vi "Top Level FPGA_w8randLED.vi"() -> ()   [LabVIEW 2012]
uses:
  <vilib>/Platform/TimedLoop/XDataNode/timing_clust.ctl
  <vilib>/Platform/TimedLoop/XDataNode/nitl_modes.ctl
  <vilib>/Platform/TimedLoop/XDataNode/wakeup.ctl
  <vilib>/rvi/DataTransferAndStorage/Container/Common/niFpgaContainerMetaDataKey.ctl
  <vilib>/rvi/DataTransferAndStorage/Container/Common/niFpgaContainerState.ctl
  <vilib>/rvi/DataTransferAndStorage/Container/Common/niFpgaDataTypeControl.ctl
  <vilib>/rvi/DataTransferAndStorage/Container/Common/niFpgaContainerImplementationControl.ctl
  <vilib>/rvi/DataTransferAndStorage/Container/Common/niFpgaContainerArbitrationOptionsControl.ctl
  <vilib>/rvi/DataTransferAndStorage/Container/Common/niFpgaTransferTypeControl.ctl
  <vilib>/rvi/DataTransferAndStorage/Container/Common/niFpgaContainerInitializationParameters.ctl
  <vilib>/rvi/Memory/Memory_Types/niFpgaMemoryInterfaceConfiguration.ctl
  <vilib>/rvi/FIFO/Fifo_Types/niFpgaFifoControlLogicControl.ctl
  <vilib>/rvi/eio/common/nirviEmuTemplateMethod_errors.vi
  <vilib>/rvi/FIFO/Fifo_Resource/nirvififoEmulationSetSize.vi
  <vilib>/rvi/DataTransferAndStorage/Container/Common/niFpgaContainerGetUniqueNameForEmu.vi
  <vilib>/rvi/Emulation/niFpgaSctlEmulationRegisterWithScheduler.vi
  <vilib>/rvi/DataTransferAndStorage/Container/Common/niFpgaContainerSetEmuInfo.vi
  <vilib>/rvi/eio/common/nirviEmuReportErrorAndStop.vi
  <vilib>/rvi/Emulation/niFpgaSctlEmulationScheduler.vi
  <vilib>/rvi/Emulation/niFpgaSctlEmulationFifoFullMgr.vi
  <vilib>/rvi/errors/niFpgaSetErrorForExecOnDevCompSimple.vi
  <vilib>/rvi/Memory/Memory_Emulation/nirvimemoryEmulationManagerCache_GetValue.vi
  <vilib>/rvi/Memory/Memory_Emulation/niFpgaMemoryEmulationValidateCache.vi
  <vilib>/rvi/Memory/Memory_Emulation/nirvimemoryEmulationManagerCache_InsertValue.vi
  <vilib>/rvi/Memory/Memory_Emulation/nirvimemoryEmulationManagerCache_SetValue.vi
  <vilib>/rvi/Emulation/niFpgaSctlEmulationResourceMgr.vi
  <vilib>/rvi/Memory/Memory_Emulation/niFpgaMemoryEmulationCacheClearOnFirstRun.vi
  <vilib>/rvi/Memory/Memory_Emulation/nirvimemoryEmulationManagerCache_MakeExclusive.vi
  <vilib>/rvi/Memory/Memory_Emulation/nirvimemoryEmulationManagerCache_ReleaseExclusive.vi
  <vilib>/Utility/error.llb/Clear Errors.vi
  <vilib>/eio/EIONode/EIONode.xnode
  <vilib>/rvi/DataTransferAndStorage/Container/XNode/niFpgaContainer.xnode
  <vilib>/rvi/FIFO/Fifo_Resource/nirvififoEmulationClear.vi
  <vilib>/Platform/TimedLoop/XDataNode/XDataNode.xnode
  <vilib>/rvi/LocalResourceManager/LocalResourceManager.xnode
  <vilib>/rvi/FIFO/Fifo_Resource/nirvififoEmulationRead.vi
  <vilib>/rvi/DataTransferAndStorage/Register/Emulation/niFpgaRegisterEmulation.vi
  <vilib>/rvi/Memory/Memory_Emulation/nirvimemoryEmulation.vi
  <vilib>/rvi/FIFO/Fifo_Resource/nirvififoEmulationWrite.vi
  <vilib>/Platform/TimedLoop/XDataNode/XDNodeRunTimeDep.lvlib
panel:
  in  "location":i16(ring) items=["Purdue", "NIKHEF", "Zurich", "???"]
  in  "Testpulse duration (20 ns ticks)":u32=5
  in  "channel 7 on/off":bool
  in  "channel 6 on/off":bool
  in  "channel 5 on/off":bool
  in  "channel 4 on/off":bool
  in  "channel 3 on/off":bool
  in  "channel 1 on/off":bool
  in  "channel 2 on/off":bool
  in  "channel 0 on/off":bool
  out "Timestamp":u64
  in  "Stop FPGA and exit":bool
  out "DMA FIFO Timed Out?":bool
  in  "Testpulser On/Off":bool
  in  "Testpulse Time Delay (20 ns ticks)":u32=14
  in  "circular buffer length":u32=1000
  in  "# of pretrigger":u32=20
  out "IO Module\\Pll Unlocked":bool
  out "IO Module\\ADC Error B":bool
  out "IO Module\\ADC Error A":bool
  out "Init Done":bool
  in  "Trigger 4":i16=4000
  in  "Trigger 5":i16=4000
  in  "Trigger 6":i16=4000
  in  "Trigger 7":i16=4000
  in  "Trigger 2":i16=4000
  in  "Trigger 3":i16=4000
  in  "Trigger 1":i16=4000
  in  "Record Size only data":u32=95
  in  "Trigger 0":i16=4000
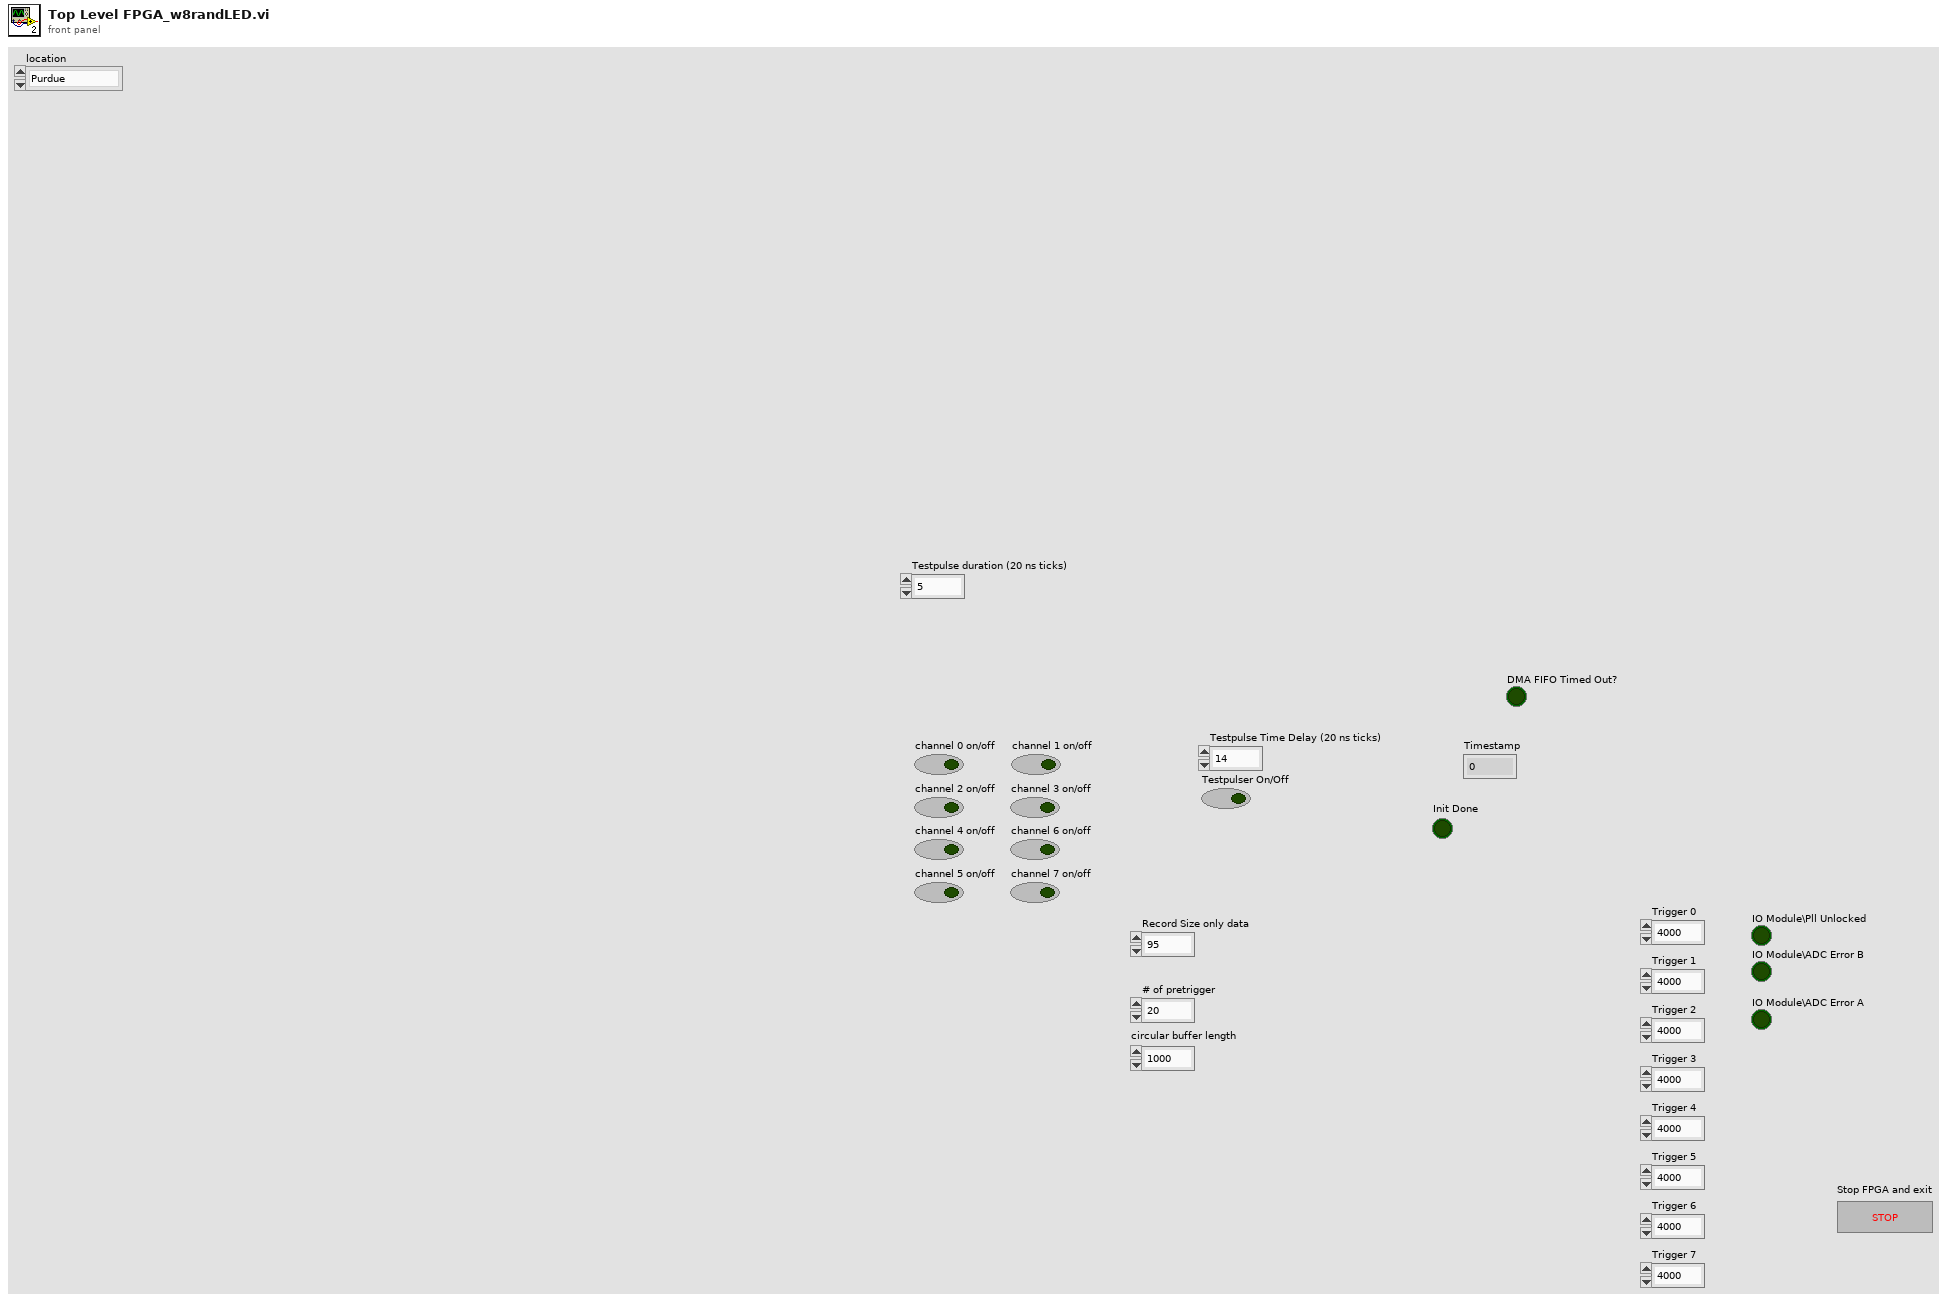
[diagram p1: front panel]
types:
  T1 = typedef "XDNodeRunTimeDep.lvlib/timing_clust.ctl" = cluster{"Expected End [f-1]":u64, "Actual End [f-1]":u64, "Finished Late? [f-1]":bool, "Expected End [i-1]":u64, "Actual End [i-1]":u64, "Finished Late? [i-1]":bool, "Expected Start [i]":u64, "Actual Start [i]":u64, "Expected Start [f]":u64, "Actual Start [f]":u64, "Source Name":string, "Structure Name":string, "Period":i64, "Deadline":i64, "Offset":i64, "Start":i64, "Priority":i32, "Timeout":i32, "Mode":T2, "Wakeup Reason":T3, "Error":errorcluster, "Source Type":string, "Secondary Source Type":string, "Global End Time":u64, "Global Start Time":u64, "Frame Duration":u64, "Iteration Duration":u64, "Assigned CPU":i32, "I/O Scan Engine Mode":u32}
  T2 = typedef "XDNodeRunTimeDep.lvlib/nitl_modes.ctl" = enum32{"No Change", "Process missed periods, maintain original phase", "Discard missed periods, maintain original phase", "Process missed periods, ignore original phase", "Discard missed periods, ignore original phase"}
  T3 = typedef "XDNodeRunTimeDep.lvlib/wakeup.ctl" = enum32{"Normal", "Aborted", "Asynchronous wakeup", "Timing source error", "Timed loop error", "Timeout"}
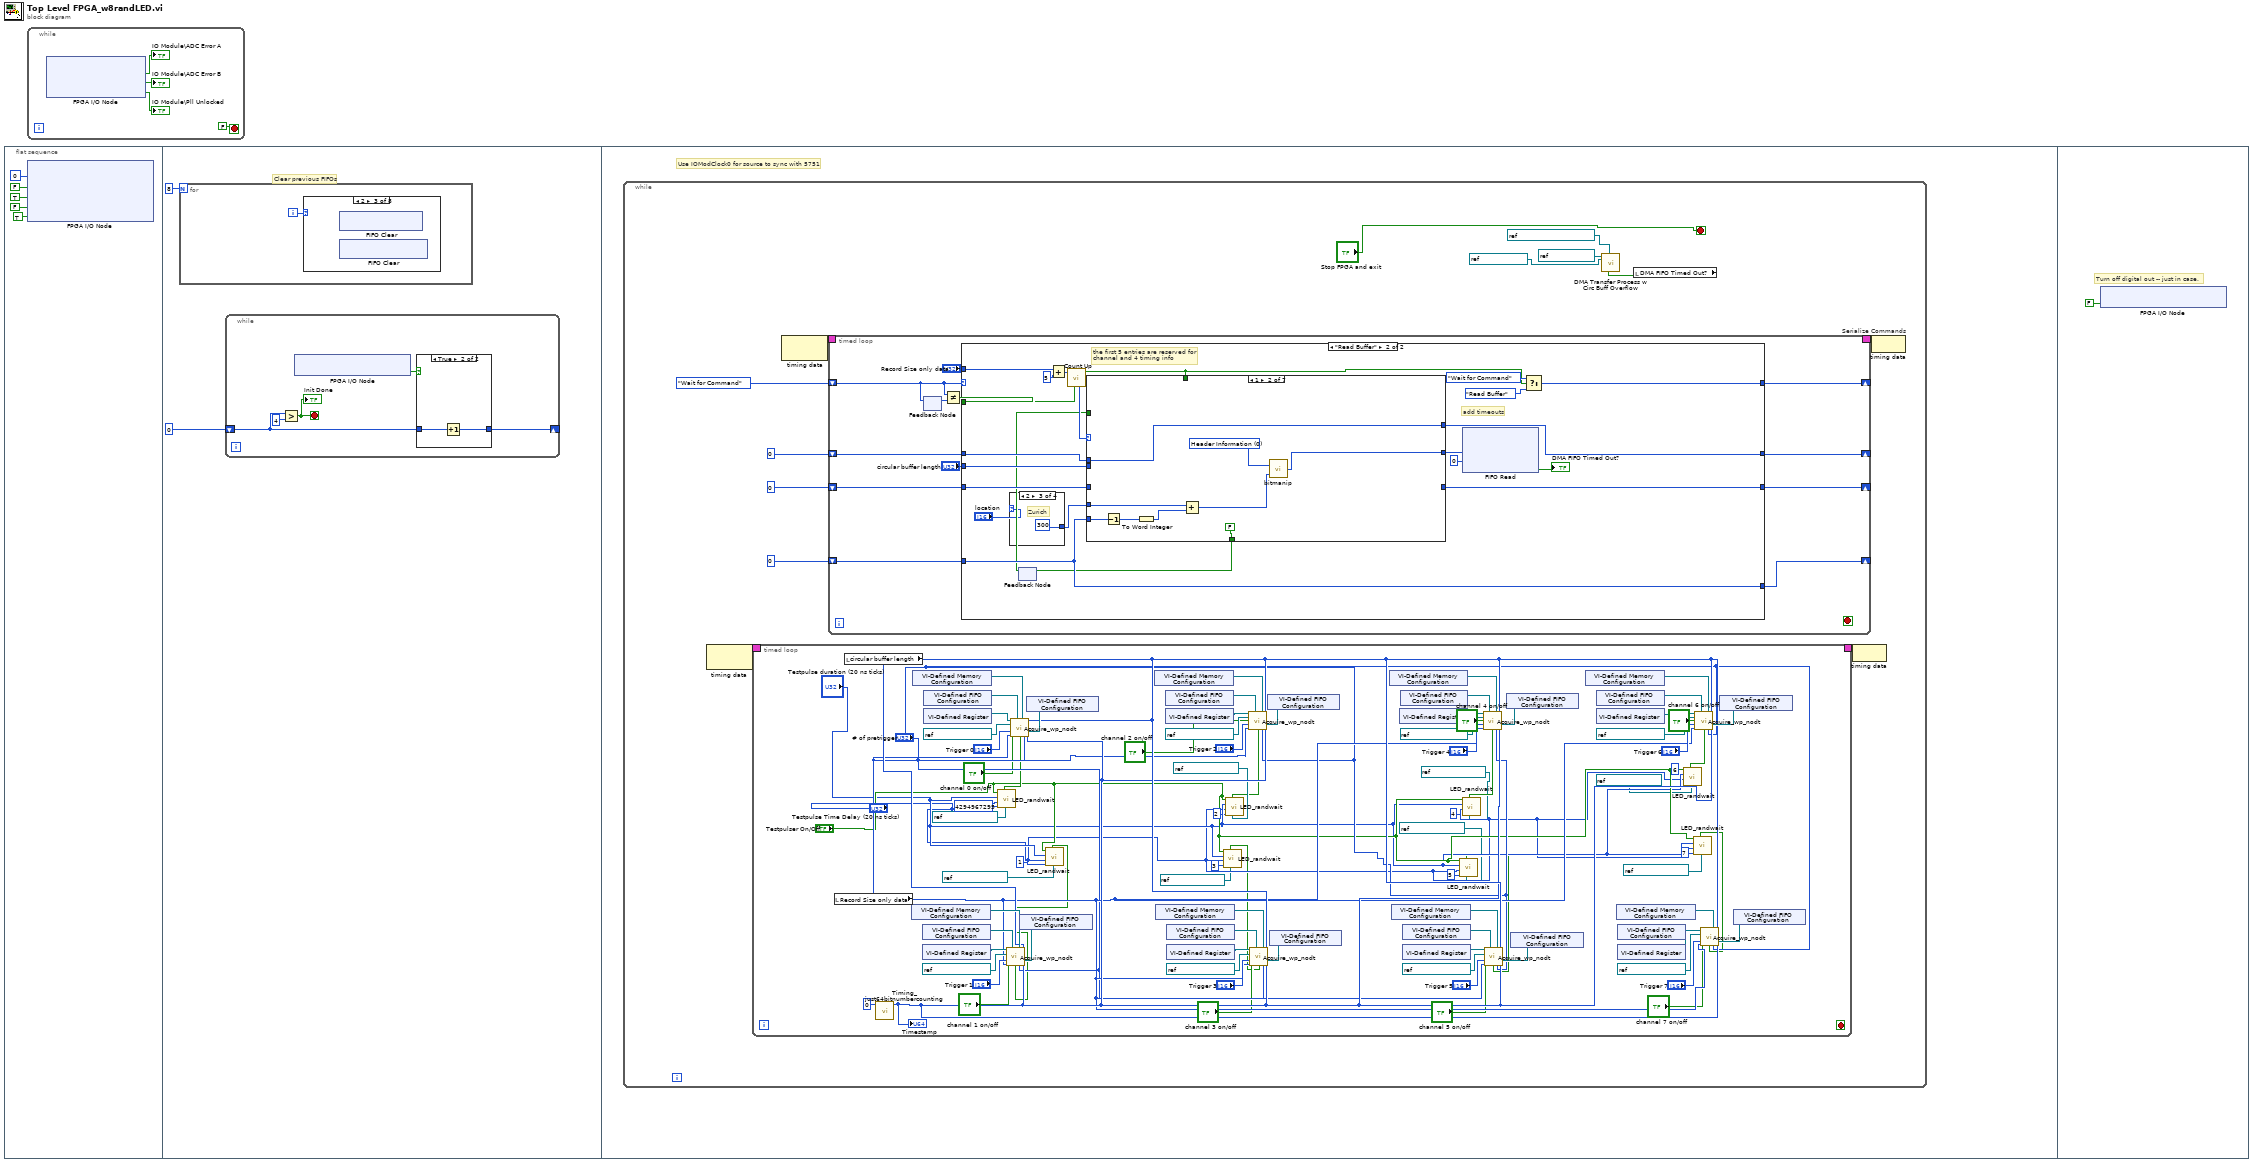
[diagram p0: block diagram]
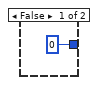
[diagram p2: hidden frame]
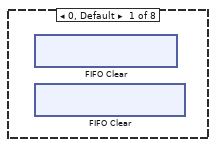
[diagram p3: hidden frame]
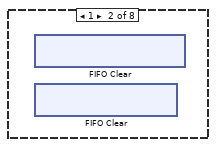
[diagram p4: hidden frame]
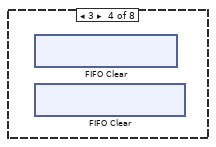
[diagram p5: hidden frame]
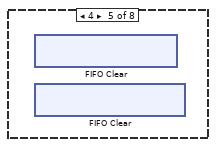
[diagram p6: hidden frame]
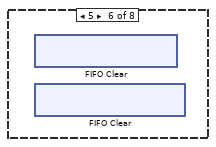
[diagram p7: hidden frame]
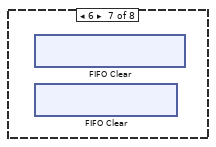
[diagram p8: hidden frame]
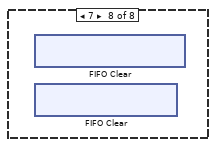
[diagram p9: hidden frame]
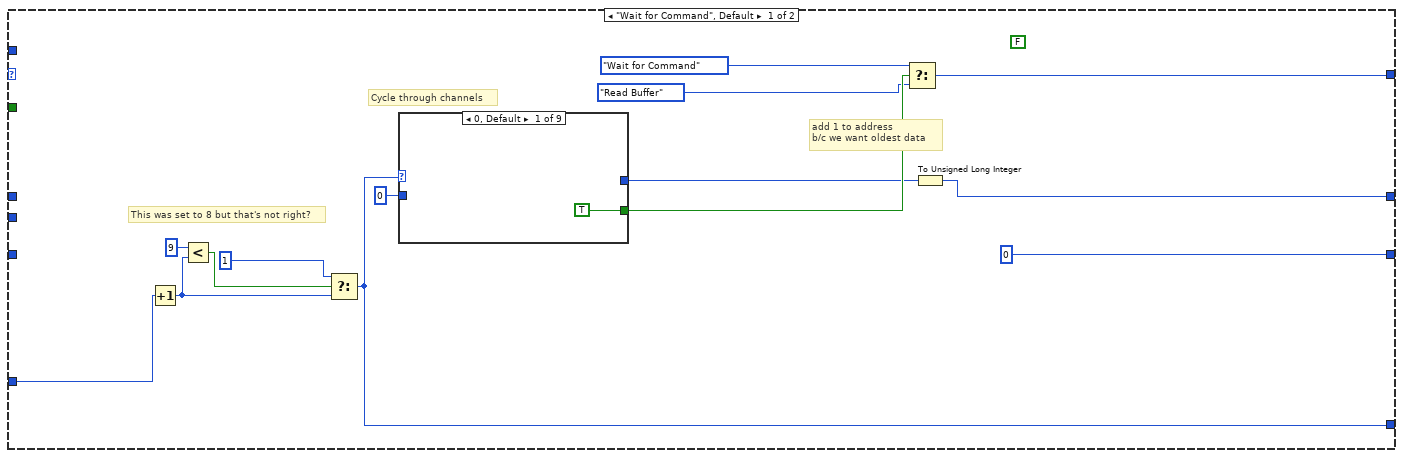
[diagram p10: hidden frame]
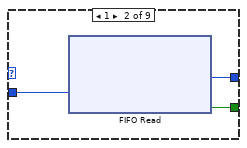
[diagram p11: hidden frame]
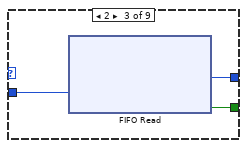
[diagram p12: hidden frame]
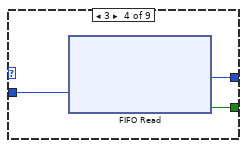
[diagram p13: hidden frame]
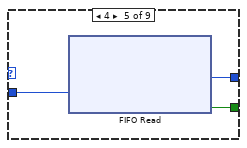
[diagram p14: hidden frame]
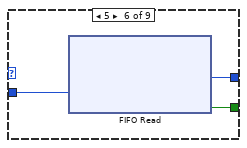
[diagram p15: hidden frame]
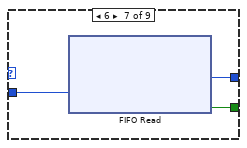
[diagram p16: hidden frame]
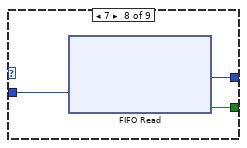
[diagram p17: hidden frame]
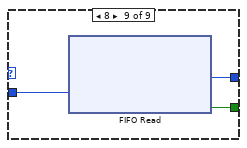
[diagram p18: hidden frame]
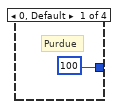
[diagram p19: hidden frame]
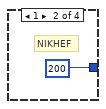
[diagram p20: hidden frame]
diagram:
  n1 = flat-sequence {
    frame #0 {
      n2 = xnode "FPGA I/O Node"("IO Module\\Sample Clock Select"=u8 0 ("IO Module\\Sample Clock Select"), "IO Module\\Force Initialization"=FALSE ("IO Module\\Force Initialization"), "IO Module\\Force Initialization"=TRUE ("IO Module\\Force Initialization"), "IO Module\\Force Initialization"=FALSE ("IO Module\\Force Initialization"), "IO Module\\Digital Output Enable"=TRUE ("IO Module\\Digital Output Enable")) -> ()  [unwired: 5 in, 5 out]
    }
    frame #1 {
      # "Clear previous FIFOs"
      n3 = for {
        N: 8 -> [_]
        i -> [w16]
        n4 = case shown="2" w16 {
          frame 0, Default {
            n5 = xnode ("FIFO Clear")() -> ()  [unwired: 1 in, 1 out]
            n6 = xnode ("FIFO Clear")() -> ()  [unwired: 1 in, 1 out]
          }
          frame 1 {
            n7 = xnode ("FIFO Clear")() -> ()  [unwired: 1 in, 1 out]
            n8 = xnode ("FIFO Clear")() -> ()  [unwired: 1 in, 1 out]
          }
          frame 2 {
            n9 = xnode ("FIFO Clear")() -> ()  [unwired: 1 in, 1 out]
            n10 = xnode ("FIFO Clear")() -> ()  [unwired: 1 in, 1 out]
          }
          frame 3 {
            n11 = xnode ("FIFO Clear")() -> ()  [unwired: 1 in, 1 out]
            n12 = xnode ("FIFO Clear")() -> ()  [unwired: 1 in, 1 out]
          }
          frame 4 {
            n13 = xnode ("FIFO Clear")() -> ()  [unwired: 1 in, 1 out]
            n14 = xnode ("FIFO Clear")() -> ()  [unwired: 1 in, 1 out]
          }
          frame 5 {
            n15 = xnode ("FIFO Clear")() -> ()  [unwired: 1 in, 1 out]
            n16 = xnode ("FIFO Clear")() -> ()  [unwired: 1 in, 1 out]
          }
          frame 6 {
            n17 = xnode ("FIFO Clear")() -> ()  [unwired: 1 in, 1 out]
            n18 = xnode ("FIFO Clear")() -> ()  [unwired: 1 in, 1 out]
          }
          frame 7 {
            n19 = xnode ("FIFO Clear")() -> ()  [unwired: 1 in, 1 out]
            n20 = xnode ("FIFO Clear")() -> ()  [unwired: 1 in, 1 out]
          }
        }
      }
      n21 = while {
        shift-right: [w11] -> _
        shift-left: u16 0 -> [w10]
        stop <- w8 stop-if-true
        n22 = Greater?(x=w10, y=u16 4) -> (0:w8:bool)
        "Init Done" <- w8
        n23 = xnode "FPGA I/O Node"() -> ("IO Module\\Initialization Done"=w12:bool)  [unwired: 1 in, 1 out]
        n24 = case shown="True" w12 {
          tunnel: [u16 0 w15] -> w11
          tunnel: w10 -> [_ w14]
          frame False {
          }
          frame True {
            n25 = Increment(x=w14) -> (x+1=w15:u16)
          }
        }
      }
    }
    frame #2 {
      # "Use IOModClock0 for source to sync with 5751"
      n26 = while {
        stop <- "Stop FPGA and exit" stop-if-true
        n27 = node-c288() -> (w22:T1)  [unwired: 1 in]
        n28 = timed-loop {
          timing: w22 -> [_]
          timing-out: [_] -> w21
          stop <- _ stop-if-true
          n29 = local read "Record Size only data"() -> (w68:u32)
          n30 = local read "circular buffer length"() -> (w70:u32)
          n31 = call "Timing_just64bitnumbercounting.vi"("initial value"=u64 0) -> ("x+1"=w69:u64)  [unwired: 10 in]
          "Timestamp" <- w69
          n32 = xnode "VI-Defined Memory Configuration"() -> ("Memory Out"=w116:refnum<k21>)
          n33 = xnode "VI-Defined Memory Configuration"() -> ("Memory Out"=w71:refnum<k21>)
          n34 = xnode "VI-Defined FIFO Configuration"() -> ("FIFO Out"=w115:refnum<k21>)
          n35 = xnode "VI-Defined Register"() -> ("Register Out"=w96:refnum<k21>)
          n36 = xnode "VI-Defined FIFO Configuration"() -> ("FIFO Out"=w72:refnum<k21>)
          n37 = xnode "VI-Defined Register"() -> ("Register Out"=w67:refnum<k21>)
          n38 = call "LED_randwait.vi"("FPGA I/O In"=refnum<k21> "IO Module\\D0 0", "seed"=u32 4294967295, "Testpulse Time Delay (20 ns ticks)"="Testpulse Time Delay (20 ns ticks)", "Testpulse duration (20 ns ticks)"="Testpulse duration (20 ns ticks)", "Testpulser On/Off"="Testpulser On/Off") -> ("Is Test Pulse?"=w56:bool)  [unwired: 5 in, 1 out]
          n39 = xnode "VI-Defined FIFO Configuration"() -> ("FIFO Out"=w82:refnum<k21>)
          n40 = xnode "VI-Defined FIFO Configuration"() -> ("FIFO Out"=w75:refnum<k21>)
          n41 = call "Acquire_wp_nodt.vi"("Ch Armed Reg"=w67, "Command FIFO"=w72, "Circular Buffer Mem"=w71, "circular buffer length"=w70, "FPGA I/O In"=refnum<k21> "IO Module\\AI A0", "channel on/off"="channel 0 on/off", "Trigger"="Trigger 0", "Timing FIFO"=w75, "Samples to Acquire"=w68, "Is Test Pulse?"=w56, "# of pretrigger"="# of pretrigger", "timing"=w69) -> ()  [unwired: 4 in]
          n42 = call "LED_randwait.vi"("FPGA I/O In"=refnum<k21> "IO Module\\D0 1", "seed"=u32 1, "Testpulse Time Delay (20 ns ticks)"="Testpulse Time Delay (20 ns ticks)", "Testpulse duration (20 ns ticks)"="Testpulse duration (20 ns ticks)", "Testpulser On/Off"="Testpulser On/Off") -> ("Is Test Pulse?"=w55:bool)  [unwired: 5 in, 1 out]
          n43 = call "Acquire_wp_nodt.vi"("Ch Armed Reg"=w96, "Command FIFO"=w115, "Circular Buffer Mem"=w116, "circular buffer length"=w70, "FPGA I/O In"=refnum<k21> "IO Module\\AI A1", "channel on/off"="channel 1 on/off", "Trigger"="Trigger 1", "Timing FIFO"=w82, "Samples to Acquire"=w68, "Is Test Pulse?"=w55, "# of pretrigger"="# of pretrigger", "timing"=w69) -> ()  [unwired: 4 in]
          n44 = xnode "VI-Defined Memory Configuration"() -> ("Memory Out"=w110:refnum<k21>)
          n45 = xnode "VI-Defined Memory Configuration"() -> ("Memory Out"=w113:refnum<k21>)
          n46 = xnode "VI-Defined FIFO Configuration"() -> ("FIFO Out"=w109:refnum<k21>)
          n47 = xnode "VI-Defined Register"() -> ("Register Out"=w92:refnum<k21>)
          n48 = xnode "VI-Defined FIFO Configuration"() -> ("FIFO Out"=w114:refnum<k21>)
          n49 = xnode "VI-Defined Register"() -> ("Register Out"=w94:refnum<k21>)
          n50 = call "LED_randwait.vi"("FPGA I/O In"=refnum<k21> "IO Module\\D0 3", "seed"=u32 3, "Testpulse Time Delay (20 ns ticks)"="Testpulse Time Delay (20 ns ticks)", "Testpulse duration (20 ns ticks)"="Testpulse duration (20 ns ticks)", "Testpulser On/Off"="Testpulser On/Off") -> ("Is Test Pulse?"=w46:bool)  [unwired: 5 in, 1 out]
          n51 = call "LED_randwait.vi"("FPGA I/O In"=refnum<k21> "IO Module\\D0 2", "seed"=u32 2, "Testpulse Time Delay (20 ns ticks)"="Testpulse Time Delay (20 ns ticks)", "Testpulse duration (20 ns ticks)"="Testpulse duration (20 ns ticks)", "Testpulser On/Off"="Testpulser On/Off") -> ("Is Test Pulse?"=w47:bool)  [unwired: 5 in, 1 out]
          n52 = xnode "VI-Defined FIFO Configuration"() -> ("FIFO Out"=w81:refnum<k21>)
          n53 = call "Acquire_wp_nodt.vi"("Ch Armed Reg"=w92, "Command FIFO"=w109, "Circular Buffer Mem"=w110, "circular buffer length"=w70, "FPGA I/O In"=refnum<k21> "IO Module\\AI A2", "channel on/off"="channel 2 on/off", "Trigger"="Trigger 2", "Timing FIFO"=w81, "Samples to Acquire"=w68, "Is Test Pulse?"=w47, "# of pretrigger"="# of pretrigger", "timing"=w69) -> ()  [unwired: 4 in]
          n54 = xnode "VI-Defined FIFO Configuration"() -> ("FIFO Out"=w80:refnum<k21>)
          n55 = call "Acquire_wp_nodt.vi"("Ch Armed Reg"=w94, "Command FIFO"=w114, "Circular Buffer Mem"=w113, "circular buffer length"=w70, "FPGA I/O In"=refnum<k21> "IO Module\\AI A3", "channel on/off"="channel 3 on/off", "Trigger"="Trigger 3", "Timing FIFO"=w80, "Samples to Acquire"=w68, "Is Test Pulse?"=w46, "# of pretrigger"="# of pretrigger", "timing"=w69) -> ()  [unwired: 4 in]
          n56 = xnode "VI-Defined Memory Configuration"() -> ("Memory Out"=w98:refnum<k21>)
          n57 = xnode "VI-Defined Memory Configuration"() -> ("Memory Out"=w101:refnum<k21>)
          n58 = xnode "VI-Defined Register"() -> ("Register Out"=w86:refnum<k21>)
          n59 = xnode "VI-Defined FIFO Configuration"() -> ("FIFO Out"=w97:refnum<k21>)
          n60 = xnode "VI-Defined FIFO Configuration"() -> ("FIFO Out"=w102:refnum<k21>)
          n61 = xnode "VI-Defined Register"() -> ("Register Out"=w90:refnum<k21>)
          n62 = call "LED_randwait.vi"("FPGA I/O In"=refnum<k21> "IO Module\\D0 5", "seed"=u32 5, "Testpulse Time Delay (20 ns ticks)"="Testpulse Time Delay (20 ns ticks)", "Testpulse duration (20 ns ticks)"="Testpulse duration (20 ns ticks)", "Testpulser On/Off"="Testpulser On/Off") -> ("Is Test Pulse?"=w44:bool)  [unwired: 5 in, 1 out]
          n63 = call "LED_randwait.vi"("FPGA I/O In"=refnum<k21> "IO Module\\D0 4", "seed"=u32 4, "Testpulse Time Delay (20 ns ticks)"="Testpulse Time Delay (20 ns ticks)", "Testpulse duration (20 ns ticks)"="Testpulse duration (20 ns ticks)", "Testpulser On/Off"="Testpulser On/Off") -> ("Is Test Pulse?"=w45:bool)  [unwired: 5 in, 1 out]
          n64 = xnode "VI-Defined FIFO Configuration"() -> ("FIFO Out"=w79:refnum<k21>)
          n65 = call "Acquire_wp_nodt.vi"("Ch Armed Reg"=w86, "Command FIFO"=w97, "Circular Buffer Mem"=w98, "circular buffer length"=w70, "FPGA I/O In"=refnum<k21> "IO Module\\AI A4", "channel on/off"="channel 4 on/off", "Trigger"="Trigger 4", "Timing FIFO"=w79, "Samples to Acquire"=w68, "Is Test Pulse?"=w45, "# of pretrigger"="# of pretrigger", "timing"=w69) -> ()  [unwired: 4 in]
          n66 = xnode "VI-Defined FIFO Configuration"() -> ("FIFO Out"=w78:refnum<k21>)
          n67 = call "Acquire_wp_nodt.vi"("Ch Armed Reg"=w90, "Command FIFO"=w102, "Circular Buffer Mem"=w101, "circular buffer length"=w70, "FPGA I/O In"=refnum<k21> "IO Module\\AI A5", "channel on/off"="channel 5 on/off", "Trigger"="Trigger 5", "Timing FIFO"=w78, "Samples to Acquire"=w68, "Is Test Pulse?"=w44, "# of pretrigger"="# of pretrigger", "timing"=w69) -> ()  [unwired: 4 in]
          n68 = xnode "VI-Defined Memory Configuration"() -> ("Memory Out"=w107:refnum<k21>)
          n69 = xnode "VI-Defined FIFO Configuration"() -> ("FIFO Out"=w108:refnum<k21>)
          n70 = xnode "VI-Defined Register"() -> ("Register Out"=w88:refnum<k21>)
          n71 = xnode "VI-Defined Memory Configuration"() -> ("Memory Out"=w104:refnum<k21>)
          n72 = xnode "VI-Defined FIFO Configuration"() -> ("FIFO Out"=w103:refnum<k21>)
          n73 = xnode "VI-Defined Register"() -> ("Register Out"=w84:refnum<k21>)
          n74 = call "LED_randwait.vi"("FPGA I/O In"=refnum<k21> "IO Module\\D0 6", "seed"=u32 6, "Testpulse Time Delay (20 ns ticks)"="Testpulse Time Delay (20 ns ticks)", "Testpulse duration (20 ns ticks)"="Testpulse duration (20 ns ticks)", "Testpulser On/Off"="Testpulser On/Off") -> ("Is Test Pulse?"=w43:bool)  [unwired: 5 in, 1 out]
          n75 = call "LED_randwait.vi"("FPGA I/O In"=refnum<k21> "IO Module\\D0 7", "seed"=u32 7, "Testpulse Time Delay (20 ns ticks)"="Testpulse Time Delay (20 ns ticks)", "Testpulse duration (20 ns ticks)"="Testpulse duration (20 ns ticks)", "Testpulser On/Off"="Testpulser On/Off") -> ("Is Test Pulse?"=w42:bool)  [unwired: 5 in, 1 out]
          n76 = xnode "VI-Defined FIFO Configuration"() -> ("FIFO Out"=w77:refnum<k21>)
          n77 = call "Acquire_wp_nodt.vi"("Ch Armed Reg"=w88, "Command FIFO"=w108, "Circular Buffer Mem"=w107, "circular buffer length"=w70, "FPGA I/O In"=refnum<k21> "IO Module\\AI A6", "channel on/off"="channel 6 on/off", "Trigger"="Trigger 6", "Timing FIFO"=w77, "Samples to Acquire"=w68, "Is Test Pulse?"=w43, "# of pretrigger"="# of pretrigger", "timing"=w69) -> ()  [unwired: 4 in]
          n78 = xnode "VI-Defined FIFO Configuration"() -> ("FIFO Out"=w76:refnum<k21>)
          n79 = call "Acquire_wp_nodt.vi"("Ch Armed Reg"=w84, "Command FIFO"=w103, "Circular Buffer Mem"=w104, "circular buffer length"=w70, "FPGA I/O In"=refnum<k21> "IO Module\\AI A7", "channel on/off"="channel 7 on/off", "Trigger"="Trigger 7", "Timing FIFO"=w76, "Samples to Acquire"=w68, "Is Test Pulse?"=w42, "# of pretrigger"="# of pretrigger", "timing"=w69) -> ()  [unwired: 4 in]
        }
        n80 = node-c288() -> (w24:T1)  [unwired: 1 in]
        n81 = timed-loop "Serialize Commands" {
          timing: w24 -> [_]
          timing-out: [_] -> w23
          shift-right: [w896] -> _
          shift-left: enum16{"Wait for Command", "Read Buffer"}."Wait for Command" -> [w894]
          shift-right: [w900] -> _
          shift-left: u32 0 ("Element") -> [w899]
          shift-right: [w898] -> _
          shift-left: u8 0 ("t") -> [w897]
          shift-right: [w891] -> _
          shift-left: u64 0 ("Element") -> [w890]
          stop <- _ stop-if-true
          n82 = feedback-in #1(w894) -> ()
          n83 = feedback #1() -> (w895:enum16{"Wait for Command", "Read Buffer"})  [unwired: 1 in]
          n84 = Not Equal?(x=w894, y=w895) -> (x != y?=w892:bool)
          n85 = case shown="\"Read Buffer\"" w894 {
            tunnel: "Record Size only data" -> [_ w951]
            tunnel: [w904 w961] -> w898
            tunnel: w897 -> [w906 w961]
            tunnel: [w907 w946] -> w900
            tunnel: w899 -> [_ w960]
            tunnel: [w910 w962] -> w896
            tunnel: "circular buffer length" -> [_ w959]
            tunnel: w892 -> [_ w953]
            tunnel: [u64 0 ("Element") w948] -> w891
            tunnel: w890 -> [_ w947]
            frame "Wait for Command", Default {
              (unwired) FALSE
              # "This was set to 8 but that's not right?"
              # "add 1 to address\nb/c we want oldest data"
              # "Cycle through channels"
              n86 = Increment(x=w906) -> (x+1=w905:u8)
              n87 = Less?(x=u8 9, y=w905) -> (x < y?=w914:bool)
              n88 = Select(t=u8 1, s=w914, f=w905) -> (s? t:f=w904:u8)
              n89 = case shown="0, Default" w904 {
                tunnel: [TRUE ("Timed Out?") w919 w920 w923 w926 w929 w932 w935 w938] -> w911
                tunnel: 0 ("Timeout") -> [_ w918 w922 w925 w928 w931 w934 w937 w940]
                tunnel: [_ w917 w921 w924 w927 w930 w933 w936 w939] -> w903
                frame 0, Default {
                }
                frame 1 {
                  n90 = xnode ("FIFO Read")("Timeout"=w918) -> ("Element"=w917:i16, "Timed Out?"=w919:bool)  [unwired: 1 in, 1 out]
                }
                frame 2 {
                  n91 = xnode ("FIFO Read")("Timeout"=w922) -> ("Element"=w921:i16, "Timed Out?"=w920:bool)  [unwired: 1 in, 1 out]
                }
                frame 3 {
                  n92 = xnode ("FIFO Read")("Timeout"=w925) -> ("Element"=w924:i16, "Timed Out?"=w923:bool)  [unwired: 1 in, 1 out]
                }
                frame 4 {
                  n93 = xnode ("FIFO Read")("Timeout"=w928) -> ("Element"=w927:i16, "Timed Out?"=w926:bool)  [unwired: 1 in, 1 out]
                }
                frame 5 {
                  n94 = xnode ("FIFO Read")("Timeout"=w931) -> ("Element"=w930:i16, "Timed Out?"=w929:bool)  [unwired: 1 in, 1 out]
                }
                frame 6 {
                  n95 = xnode ("FIFO Read")("Timeout"=w934) -> ("Element"=w933:i16, "Timed Out?"=w932:bool)  [unwired: 1 in, 1 out]
                }
                frame 7 {
                  n96 = xnode ("FIFO Read")("Timeout"=w937) -> ("Element"=w936:i16, "Timed Out?"=w935:bool)  [unwired: 1 in, 1 out]
                }
                frame 8 {
                  n97 = xnode ("FIFO Read")("Timeout"=w940) -> ("Element"=w939:i16, "Timed Out?"=w938:bool)  [unwired: 1 in, 1 out]
                }
              }
              n98 = Select(t=enum16{"Wait for Command", "Read Buffer"}."Wait for Command", s=w911, f=enum16{"Wait for Command", "Read Buffer"}."Read Buffer") -> (s? t:f=w910:enum16{"Wait for Command", "Read Buffer"})
              n99 = To Unsigned Long Integer(number=w903) -> (unsigned 32bit integer=w907:u32)
            }
            frame "Read Buffer" {
              # "the first 5 entries are reserved for channel and 4 timing info"
              # "add timeouts"
              n100 = case shown="2" "location" {
                tunnel: [i16 100 i16 200 i16 300 i16 400] -> w941
                frame 0, Default {
                  # "Purdue"
                }
                frame 1 {
                  # "NIKHEF"
                }
                frame 2 {
                  # "Zurich"
                }
                frame 3 {
                  # "???"
                }
              }
              n101 = feedback #2() -> (w945:bool)  [unwired: 1 in]
              n102 = Add(x=w951, y=u32 5) -> (x+y=w949:u32)
              n103 = call "Count Up.vi"("Reset?"=w953, "goal"=w949) -> ("Count Met"=w955:bool, "count"=w952:u32)  [unwired: 8 in]
              n104 = case shown="1" w952 {
                tunnel: w961 -> [_ w974 w982 _ _ _ w1021]
                tunnel: w960 -> [_ w979 w984 w1005 w1011 w1017 w1028]
                tunnel: w959 -> [_ _ _ _ _ _ w1027]
                tunnel: w955 -> [_ _ _ _ _ _ w1026]
                tunnel: [i16 0 ("Data") w977 w986 w1003 w1009 w1015 w1022] -> w954
                tunnel: w945 -> [_ _ _ _ _ _ w1024]
                tunnel: [u64 0 ("Element") _ w983 w1006 w1012 w1018 _] -> w948
                tunnel: w947 -> [_ _ _ w1006 w1012 w1018 _]
                tunnel: [u32 0 ("Element") w979 w984 w1005 w1011 w1017 _] -> w946
                tunnel: [FALSE FALSE FALSE FALSE FALSE TRUE FALSE] -> w944
                tunnel: w941 -> [_ w972 _ _ _ _ _]
                frame 0, Default {
                }
                frame 1 {
                  w976 = u16 0 items=["Header Information", "Particle Pulse", "Test Pulse"] ("Pulse Type")
                  n105 = Decrement(x=w974) -> (x-1=w975:u8)
                  n106 = To Word Integer(number=w975) -> (16bit integer=w973:i16)
                  n107 = Add(x=w972, y=w973) -> (x+y=w971:i16)
                  n108 = call "bitmanip.vi"("Pulse Type"=w976, "Integer to be written"=w971) -> ("Integer Written"=w977:i16)  [unwired: 2 in]
                }
                frame 2 {
                  # "reads out the lsb of the timing information"
                  n109 = case shown="2" w982 {
                    tunnel: [_ w987 w989 w991 w993 w995 w997 w999 w1001] -> w983
                    frame Default {
                    }
                    frame 1 {
                      n110 = xnode ("FIFO Read")("Timeout"=0) -> ("Element"=w987:u64)  [unwired: 1 in, 2 out]
                    }
                    frame 2 {
                      n111 = xnode ("FIFO Read")("Timeout"=0) -> ("Element"=w989:u64)  [unwired: 1 in, 2 out]
                    }
                    frame 3 {
                      n112 = xnode ("FIFO Read")("Timeout"=0) -> ("Element"=w991:u64)  [unwired: 1 in, 2 out]
                    }
                    frame 4 {
                      n113 = xnode ("FIFO Read")("Timeout"=0) -> ("Element"=w993:u64)  [unwired: 1 in, 2 out]
                    }
                    frame 5 {
                      n114 = xnode ("FIFO Read")("Timeout"=0) -> ("Element"=w995:u64)  [unwired: 1 in, 2 out]
                    }
                    frame 6 {
                      n115 = xnode ("FIFO Read")("Timeout"=0) -> ("Element"=w997:u64)  [unwired: 1 in, 2 out]
                    }
                    frame 7 {
                      n116 = xnode ("FIFO Read")("Timeout"=0) -> ("Element"=w999:u64)  [unwired: 1 in, 2 out]
                    }
                    frame 8 {
                      n117 = xnode ("FIFO Read")("Timeout"=0) -> ("Element"=w1001:u64)  [unwired: 1 in, 2 out]
                    }
                  }
                  n118 = Split Number(x=w983) -> (hi(x)=w981:u32)  [unwired: 1 out]
                  n119 = Split Number(x=w981) -> (hi(x)=w980:u16)  [unwired: 1 out]
                  n120 = To Word Integer(number=w980) -> (16bit integer=w986:i16)
                }
                frame 3 {
                  n121 = Split Number(x=w1006) -> (hi(x)=w1008:u32)  [unwired: 1 out]
                  n122 = Split Number(x=w1008) -> (lo(x)=w1007:u16)  [unwired: 1 out]
                  n123 = To Word Integer(number=w1007) -> (16bit integer=w1003:i16)
                }
                frame 4 {
                  n124 = Split Number(x=w1012) -> (lo(x)=w1014:u32)  [unwired: 1 out]
                  n125 = Split Number(x=w1014) -> (hi(x)=w1013:u16)  [unwired: 1 out]
                  n126 = To Word Integer(number=w1013) -> (16bit integer=w1009:i16)
                }
                frame 5 {
                  n127 = Split Number(x=w1018) -> (lo(x)=w1020:u32)  [unwired: 1 out]
                  n128 = Split Number(x=w1020) -> (lo(x)=w1019:u16)  [unwired: 1 out]
                  n129 = To Word Integer(number=w1019) -> (16bit integer=w1015:i16)
                }
                frame 6.. {
                  n130 = call "Circular Buffer Address_try_without_deadtime.vi"("Reset?"=w1024, "Starting Address"=w1028, "circular buffer length"=w1027) -> ("Address"=w1025:u32)  [unwired: 8 in]
                  n131 = case shown="1" w1021 {
                    tunnel: w1025 -> [_ w1032 w1035 w1038 w1041 w1044 w1047 w1050 w1053]
                    tunnel: w1026 -> [_ w1031 w1034 w1037 w1040 w1043 w1046 w1049 w1052]
                    tunnel: [i16 0 w1030 w1033 w1036 w1039 w1042 w1045 w1048 w1051] -> w1022
                    frame Default {
                      # "Error"
                    }
                    frame 1 {
                      n132 = xnode ("Memory Read")("Address"=w1032) -> ("Data"=w1030:i16)  [unwired: 1 in, 1 out]
                      n133 = xnode ("Register Write")("Data"=w1031) -> ()  [unwired: 1 in, 1 out]
                    }
                    frame 2 {
                      n134 = xnode ("Memory Read")("Address"=w1035) -> ("Data"=w1033:i16)  [unwired: 1 in, 1 out]
                      n135 = xnode ("Register Write")("Data"=w1034) -> ()  [unwired: 1 in, 1 out]
                    }
                    frame 3 {
                      n136 = xnode ("Memory Read")("Address"=w1038) -> ("Data"=w1036:i16)  [unwired: 1 in, 1 out]
                      n137 = xnode ("Register Write")("Data"=w1037) -> ()  [unwired: 1 in, 1 out]
                    }
                    frame 4 {
                      n138 = xnode ("Memory Read")("Address"=w1041) -> ("Data"=w1039:i16)  [unwired: 1 in, 1 out]
                      n139 = xnode ("Register Write")("Data"=w1040) -> ()  [unwired: 1 in, 1 out]
                    }
                    frame 5 {
                      n140 = xnode ("Memory Read")("Address"=w1044) -> ("Data"=w1042:i16)  [unwired: 1 in, 1 out]
                      n141 = xnode ("Register Write")("Data"=w1043) -> ()  [unwired: 1 in, 1 out]
                    }
                    frame 6 {
                      n142 = xnode ("Memory Read")("Address"=w1047) -> ("Data"=w1045:i16)  [unwired: 1 in, 1 out]
                      n143 = xnode ("Register Write")("Data"=w1046) -> ()  [unwired: 1 in, 1 out]
                    }
                    frame 7 {
                      n144 = xnode ("Memory Read")("Address"=w1050) -> ("Data"=w1048:i16)  [unwired: 1 in, 1 out]
                      n145 = xnode ("Register Write")("Data"=w1049) -> ()  [unwired: 1 in, 1 out]
                    }
                    frame 8 {
                      n146 = xnode ("Memory Read")("Address"=w1053) -> ("Data"=w1051:i16)  [unwired: 1 in, 1 out]
                      n147 = xnode ("Register Write")("Data"=w1052) -> ()  [unwired: 1 in, 1 out]
                    }
                  }
                }
              }
              n148 = feedback-in #2(w944) -> ()
              n149 = xnode ("FIFO Read")("Element"=w954, "Timeout"=0) -> ("Timed Out?"=→"DMA FIFO Timed Out?":bool)  [unwired: 1 in, 1 out]
              n150 = Select(t=enum16{"Wait for Command", "Read Buffer"}."Wait for Command", s=w955, f=enum16{"Wait for Command", "Read Buffer"}."Read Buffer") -> (s? t:f=w962:enum16{"Wait for Command", "Read Buffer"})
            }
          }
        }
        n151 = local read "DMA FIFO Timed Out?"() -> (w27:bool)
        n152 = call "DMA Transfer Process w Circ Buff Overflow.vi"("DMA Write Timed Out?"=w27, "Clock Domain"=refnum<k21> "40 MHz Onboard Clock", "Local"=refnum<k21> "To DMA FIFO", "DMA"=refnum<k21> "To Host FIFO") -> ()  [unwired: 8 in]
        n153 = node-c288(w21) -> ()
        n154 = node-c288(w23) -> ()
      }
    }
    frame #3 {
      # "Turn off digital out -- just in case."
      n155 = xnode "FPGA I/O Node"("IO Module\\Digital Output Enable"=FALSE ("IO Module\\Digital Output Enable")) -> ()  [unwired: 1 in, 1 out]
    }
  }
  n156 = while {
    stop <- FALSE stop-if-true
    n157 = xnode "FPGA I/O Node"() -> ("IO Module\\ADC Error A"=→"IO Module\\ADC Error A":bool, "IO Module\\ADC Error B"=→"IO Module\\ADC Error B":bool, "IO Module\\Pll Unlocked"=→"IO Module\\Pll Unlocked":bool)  [unwired: 3 in, 3 out]
  }
